vi "PCO_GetTriggerMode.vi"(8 "error in (no error)":errorcluster {"code" format="%x"}, 11 "ph":u64) -> (0 "error out":errorcluster {"code" format="%x"}, 1 "wTriggerMode":u16(ring) items=["auto sequence"=0, "software trigger"=1, "external exposure start & software trigger"=2, "external exposure control"=3, "external synchronized"=4, "fast external exposure control"=5, "external CDS control"=6, "slow external exposure control"=7, "external synchronized HDSDI"=258], 2 "ErrorMessage":i32 format="%x", 3 "ph out":u64)   [LabVIEW 2019, in "SDK.lvlib" / "TimingControl.lvlib"]
doc: "<b>Description:</b>\nThis function returns the current trigger mode setting of the camera.\nDetailed description of trigger and acquire modes can be found in the respective camera manual.\nIn all trigger modes effective image exposure depends also on the acquire mode settings and the acquire signal input.\n\n<b>Supported camera type:</b>\nAll cameras\n\n<b>Descriptor dependency:</b>\nNone"
uses:
  TimingControl.lvlib
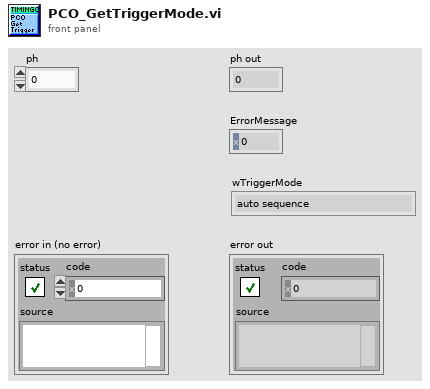
[diagram p1: front panel]
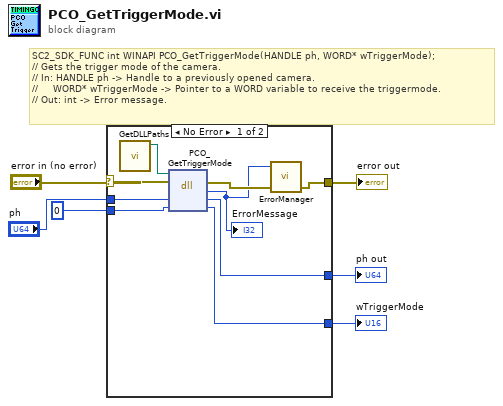
[diagram p0: block diagram]
diagram:
  # "SC2_SDK_FUNC int WINAPI PCO_GetTriggerMode(HANDLE ph, WORD* wTriggerMode);\n// Gets the trigger mode of the camera.\n// In: HANDLE ph -> Handle to a previously opened camera.\n//     WORD* wTriggerMode -> Pointer to a WORD variable to receive the triggermode.\n// Out: int -> Error message."
  n1 = case shown="No Error" "error in (no error)" {
    selector: "error in (no error)" -> [w11 w18]
    tunnel: "ph" -> [w15 w17]
    tunnel: [w14 w17] -> w5
    tunnel: u16 0 ("wTriggerMode") -> [w13 w16]
    tunnel: [w12 w16] -> w3
    tunnel: [w9 w18] -> w2
    frame No Error {
      n2 = call "GetDLLPaths.vi"() -> ("SC2_Cam_Path"=w7:path)  [unwired: 9 in, 2 out]
      n3 = dll-call lib="?" fn="PCO_GetTriggerMode"(path in=w7, error in=w11, "ph"=w15, "wTriggerMode"=w13) -> (error out=w10:errorcluster, "return type"=w8:i32, "ph"=w14:u64, "wTriggerMode"=w12:u16)  [unwired: 1 in, 1 out]
      "ErrorMessage" <- w8
      n4 = call "ErrorManager.vi"("error in (no error)"=w10, "error code"=w8) -> ("error out"=w9:errorcluster)  [unwired: 3 in]
    }
    frame Error {
    }
  }
  "ph out" <- w5
  "wTriggerMode" <- w3
  "error out" <- w2
